vi "Get_Time_Power_Required.vi"(0 "Recipe_Data_Dispaly":string[][](array[string]), 5 "Recipe_Code":i32, 9 "Current_Stage":i32) -> (4 "Time_Required":dbl, 6 "Power_Required":i32)   [LabVIEW 2021]
doc: "Used to get the power and time required to cook the recipe from the data base"
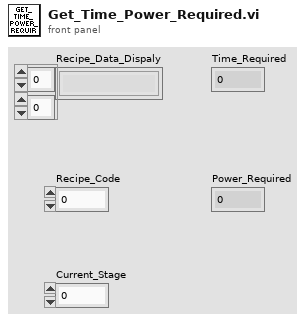
[diagram p1: front panel]
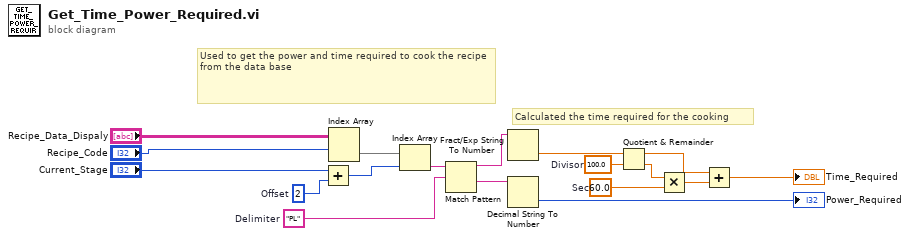
[diagram p0: block diagram]
diagram:
  w10 = 60.0  # Sec
  w9 = 100.0  # Divisor
  w4 = "PL"  # Delimiter
  w3 = 2  # Offset
  # "Calculated the time required for the cooking"
  # "Used to get the power and time required to cook the recipe from the data base"
  n1 = Add(x="Current_Stage", y=w3) -> (x+y=w15:i32)
  n2 = Index Array(array="Recipe_Data_Dispaly", index (row)="Recipe_Code") -> (element=w2:string[])  [unwired: 1 in]
  n3 = Index Array(array=w2, index=w15) -> (element=w14:string)
  n4 = Match Pattern(string=w14, regular expression=w4) -> (before substring=w7:string, after substring=w5:string)  [unwired: 1 in, 2 out]
  n5 = Fract/Exp String To Number(string=w7) -> (number=w8:dbl)  [unwired: 3 in, 1 out]
  n6 = Decimal String To Number(string=w5) -> (number=→"Power_Required":i32)  [unwired: 2 in, 1 out]
  n7 = Quotient & Remainder(x=w8, y=w9) -> (x-y*floor(x/y)=w12:dbl, floor(x/y)=w13:dbl)
  n8 = Multiply(x=w13, y=w10) -> (x*y=w11:dbl)
  n9 = Add(x=w12, y=w11) -> (x+y=→"Time_Required":dbl)
